vi "U6 Quadrature 2-Input.vi"(8 "error in":errorcluster) -> (0 "error out":errorcluster)   [LabVIEW 2021]
panel:
  out "Quadrature Count 2/3":i32
  in  "Stop":bool
  in  "Reset Count":bool
  out "Quadrature Count 0/1":i32
  in  "FirstFound":bool=TRUE
  in  "Address":string="1"
  out "Error Message":string
  # "Demonstrates 2 quadrature inputs.  The first uses Timer0/Timer1 on FIO0/FIO1 for phases A & B.  The\nsecond uses Timer2/Timer3 on FIO2/FIO3 for phases A & B.\n\nIf you don't have a quadrature signal source handy, you can connect wires to GND, and tap these wires on FIO0/FIO1\nor FIO2/FIO3 to roughly simulate quadrature."
  # "This VI passes a timer\nbase clock constant that\nis valid for hardware V1.21.\nFor hardware V1.20 change\nLJ_tc48MHZ to LJ_tc24MHZ."
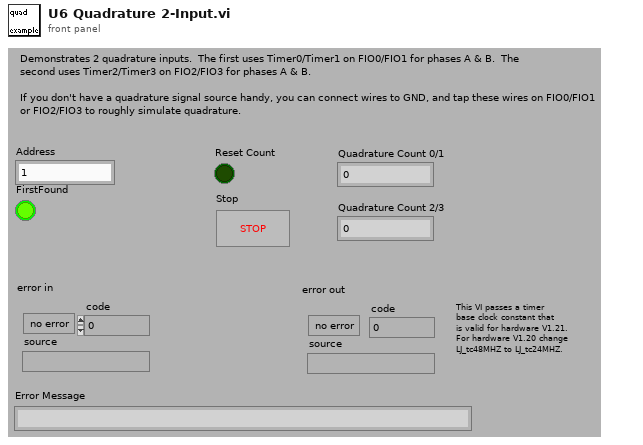
[diagram p1: front panel]
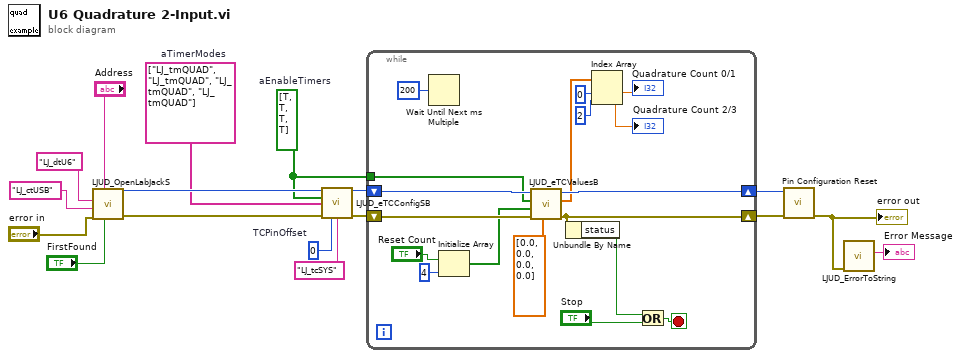
[diagram p0: block diagram]
diagram:
  w2 = 0  # TCPinOffset
  w1 = bool[] [TRUE, TRUE, TRUE, TRUE]  # aEnableTimers
  w4 = string[] ["LJ_tmQUAD", "LJ_tmQUAD", "LJ_tmQUAD", "LJ_tmQUAD"]  # aTimerModes
  n1 = call "LJUD_OpenLabJackS.vi"("FirstFound"="FirstFound", "Address"="Address", "error in"="error in", "ConnectionType"="LJ_ctUSB", "DeviceType"="LJ_dtU6") -> ("error out"=w8:errorcluster, "Handle"=w7:i32)  [unwired: 4 in, 1 out]
  n2 = call "LJUD_eTCConfigSB.vi"("Handle In"=w7, "aEnableTimers"=w1, "aTimerModes"=w4, "error in"=w8, "TCPinOffset"=w2, "TimerClockBase"="LJ_tcSYS") -> ("Handle Out"=w5:i32, "error out"=w6:errorcluster)  [unwired: 8 in]
  n3 = while {
    tunnel: w1 -> [w21]
    shift-left: w6 -> [w23]
    shift-right: [w33] -> w10
    shift-left: w5 -> [w24]
    shift-right: [w26] -> w11
    stop <- w32 stop-if-true
    n4 = Wait Until Next ms Multiple(millisecond multiple=u32 200) -> ()  [unwired: 1 out]
    n5 = Initialize Array("Reset Count", 4 ("Dimension Size")) -> (w20:bool[])
    n6 = call "LJUD_eTCValuesB.vi"("aTimerValues Write"=dbl[] [0.0, 0.0, 0.0, 0.0], "error in"=w23, "aUpdateResetTimers"=w20, "aReadTimers"=w21, "Handle In"=w24) -> ("error out"=w33:errorcluster, "aTimerValues Read"=w25:dbl[], "Handle Out"=w26:i32)  [unwired: 3 in, 1 out]
    n7 = Unbundle By Name(w33) -> ("status"=w31:bool)
    n8 = Index Array(array=w25, index #1=0 ("Index"), index #2=2 ("Index")) -> (element #1=→"Quadrature Count 0/1":dbl, element #2=→"Quadrature Count 2/3":dbl)
    n9 = Or(x=w31, y="Stop") -> (x .or. y?=w32:bool)
  }
  n10 = call "Pin Configuration Reset.vi"("error in"=w10, "Handle In"=w11) -> ("error out"=w9:errorcluster)  [unwired: 8 in, 1 out]
  "error out" <- w9
  n11 = call "LJUD_ErrorToString.vi"("error in"=w9) -> ("String"=→"Error Message":string)  [unwired: 10 in]
